vi "Initialize Work.vi"(8 "error in (no error)":errorcluster, 9 "Update period":dbl, 10 "Reply to":refnum<class "Result Reply Msg.lvclass">, 11 "Measure Object in":refnum<class "Simple Sequencer.lvclass">) -> (0 "error out":errorcluster, 3 "Measure Object out":refnum<class "Simple Sequencer.lvclass">)   [LabVIEW 2018, in "Simple Sequencer.lvclass"]
uses:
  Simple Sequencer.lvclass
  Template Module Messages/Result Reply Msg/Result Reply Msg.lvclass
  Worker/Worker.lvclass
  NHMFL_Core/Libraries/Instruments/Sequence/Sequencer State Machine/Sequencer State Machine.lvclass
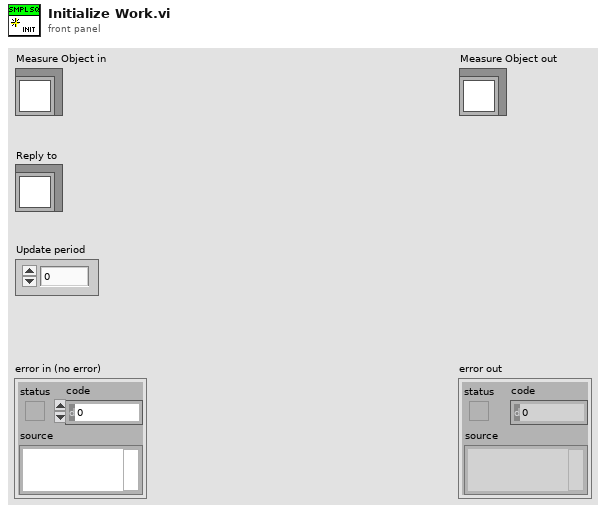
[diagram p1: front panel]
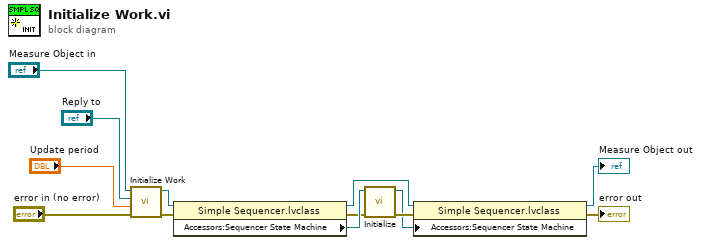
[diagram p0: block diagram]
diagram:
  n1 = call-parent "Initialize Work.vi"("error in (no error)"="error in (no error)", "Update period"="Update period", "Reply to"="Reply to", "Measure Object in"="Measure Object in") -> ("error out"=w13:errorcluster, "Measure Object out"=w8:refnum<class "Simple Sequencer.lvclass">)  [unwired: 6 in]
  n2 = property class="Simple Sequencer.lvclass"(reference=w8, error in=w13) -> (reference out=w2:refnum<class "Simple Sequencer.lvclass">, error out=w6:errorcluster, "Accessors:Sequencer State Machine"=w7:refnum<class "Sequencer State Machine.lvclass">)
  n3 = call-dynamic "Initialize.vi"("error in (no error)"=w6, "Sequencer State Machine in"=w7) -> ("error out"=w5:errorcluster, "Sequencer State Machine out"=w4:refnum<class "Sequencer State Machine.lvclass">)  [unwired: 8 in]
  n4 = property class="Simple Sequencer.lvclass"(reference=w2, error in=w5, "Accessors:Sequencer State Machine"=w4) -> (reference out=→"Measure Object out":refnum<class "Simple Sequencer.lvclass">, error out=→"error out":errorcluster)
